vi "Mouse In.vi"(8 "error in (no error)":errorcluster, 10 "MousePoint":cluster{"x":i16, "y":i16}, 11 "Line Border in":refnum<class "Line Border.lvclass">) -> (0 "error out":errorcluster, 2 "In?":bool, 3 "Line Border out":refnum<class "Line Border.lvclass">)   [LabVIEW 2015, in "Line Border.lvclass"]
uses:
  Line Border.lvclass
  Scalable Border/Scalable Border.lvclass/Scalable Border.ctl
  Scalable Border/Scalable Border.lvclass
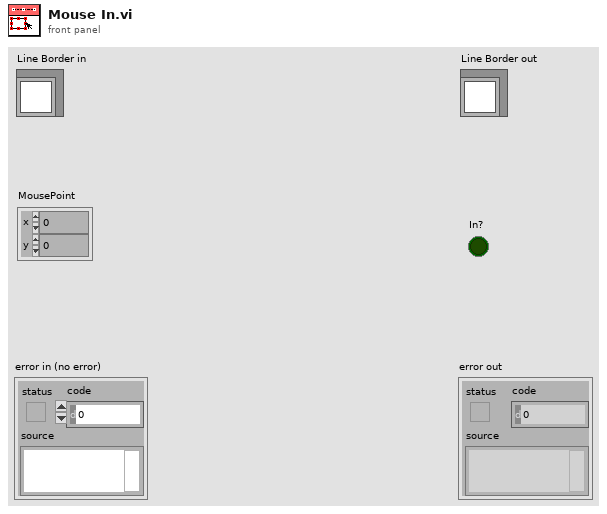
[diagram p1: front panel]
types:
  T1 = cluster{"left":i16, "top":i16, "right":i16, "bottom":i16}[]
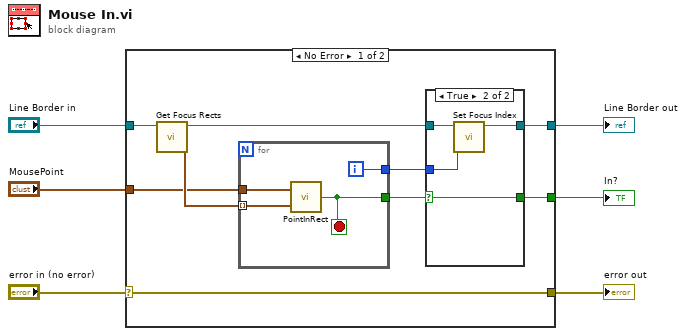
[diagram p0: block diagram]
diagram:
  n1 = case shown="No Error" "error in (no error)" {
    selector: "error in (no error)" -> [w15 w27]
    tunnel: "Line Border in" -> [w14 w26]
    tunnel: "MousePoint" -> [w11 _]
    tunnel: [w10 w26] -> w3
    tunnel: [w7 _] -> w2
    tunnel: [w15 w27] -> w1
    frame No Error {
      n2 = call "Get Focus Rects.vi"("Scalable Border in"=w14) -> ("Focus Rects"=w12:T1, "Scalable Border out"=w13:refnum<class "Line Border.lvclass">)  [unwired: 8 in, 1 out]
      n3 = for {
        tunnel: w12 -> [w25] mode=indexing
        tunnel: w11 -> [w24]
        tunnel: [w23] -> w9
        tunnel: [w22] -> w8
        i -> [w23]
        stop <- w22 stop-if-true
        n4 = call <vilib>:"PointInRect.vi"("rect"=w25, "point"=w24) -> ("pt in rect"=w22:bool)
      }
      n5 = case shown="True" w8 {
        selector: w8 -> [w16 w18]
        tunnel: w13 -> [w17 w21]
        tunnel: [w17 w20] -> w10
        tunnel: w9 -> [_ w19]
        tunnel: [w16 w18] -> w7
        frame False {
        }
        frame True {
          n6 = call "Set Focus Index.vi"("Focus Index"=w19, "Scalable Border in"=w21) -> ("Scalable Border out"=w20:refnum<class "Line Border.lvclass">)  [unwired: 8 in, 1 out]
        }
      }
    }
    frame Error {
    }
  }
  "error out" <- w1
  "Line Border out" <- w3
  "In?" <- w2
